vi "Experimental Flat-line Signal.vi"(1 "Flatline Offset":dbl format="%0.2p") -> (0 "Flatline Signal":waveform(dbl))   [LabVIEW 2013]
uses:
  <vilib>/measure/NI_MABase.lvlib
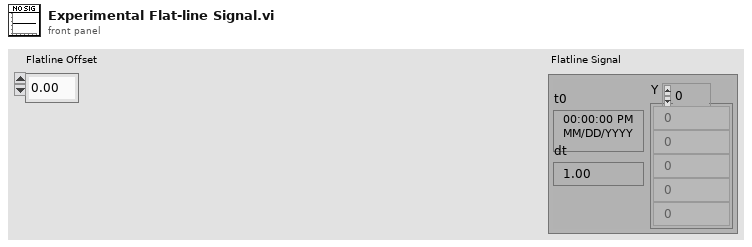
[diagram p1: front panel]
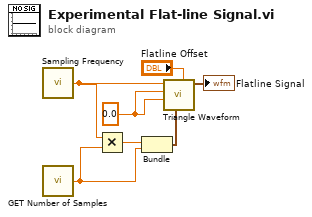
[diagram p0: block diagram]
diagram:
  w5 = 0.0 ("amplitude")
  n1 = call "Sampling Frequency.vi"() -> ("Sampling Frequency"=w1:dbl)
  n2 = call "GET Number of Samples.vi"() -> ("Number of Samples"=w3:dbl)
  n3 = Multiply(x=w1, y=w3) -> (x*y=w4:dbl)
  n4 = Bundle(w4, "Number of Samples"=w3) -> (w2:cluster{dbl, "Number of Samples":dbl})  [unwired: 1 in]
  n5 = call <vilib>:"Triangle Waveform.vi"("offset"="Flatline Offset", "sampling info"=w2, "phase"=w5, "amplitude"=w5, "frequency"=w1) -> ("signal out"=→"Flatline Signal":waveform(dbl))  [unwired: 5 in, 1 out]
